vi "Heater Main PID.vi"() -> ()   [LabVIEW 2019]
doc: "This example demonstrates how to acquire a continuous amount of data (Waveform) using the DAQ device's internal clock. It also shows how to synchronize two devices for different device families (E Series, S Series, M Series, X Series, DSA, and SC Express), to simultaneously acquire the data.\n\nFor instructions on how to connect your signals to the DAQ device, refer to your device documentation."
uses:
  <vilib>/Utility/error.llb/DialogType.ctl
  <vilib>/DAQmx/write.llb/DAQmx Write (Analog DBL 1Chan 1Samp).vi
  <vilib>/DAQmx/read.llb/DAQmx Read (Analog 1D Wfm NChan NSamp).vi
  <vilib>/DAQmx/configure/timing.llb/DAQmx Timing (Sample Clock).vi
  <vilib>/DAQmx/miscellaneous.llb/DAQmx Fill In Error Info.vi
  <vilib>/addons/control/pid/pid.llb/PID (DBL).vi
  <vilib>/addons/control/pid/NI_PID_pid.lvlib
panel:
  in  "Microhotplate Logger":T1(tab)
  in  "Stop":bool
  in  "Enable logging":bool caption="Enable"
  in  "File config":T2={"Filepath"=path "C:/Users/Administrator/Desktop/DAQ Heater Control/Test data", "Test ID"="test", "PC"="69DTQV2"}
  in  "Sampling config":cluster{"Fs":dbl, "#s":dbl}={"Fs"=1000.0, "#s"=1000.0} {"Fs" format="%.2p"}
  out "Logging":bool=TRUE
  in  "Output channel config":T3={"Output channel"="Dev1/ao0", "name to assign"="Heater Voltage"}
  in  "Voltage output limit":dbl=3.0 caption="Amplitude"
  in  "Current channel config":T4={"Channel Index"=1, "Shunt resistance"=10.0, "Channel name"="Heater Current"} {"Shunt resistance" format="%.4f"}
  in  "IV channel config":T5={"Voltage channel index"=0, "Current channel index"=2}
  out "IV channel names":T6={"Voltage channel name"="Heater Voltage", "Current channel name"="Heater Current"}
  in  "TCR config":T7={"TCR1"=0.00205, "TCR2"=3e-07, "TRH"=0.766, "TRM"=0.928} {"TRM" format="%.3f"; "TRH" format="%.3f"; "TCR2" format="%.2e"; "TCR1" format="%.2e"}
  in  "Ramb config":cluster{"Tamb":dbl, "Ramb":dbl}={"Tamb"=25.0, "Ramb"=39.041} {"Ramb" format="%.3f"; "Tamb" format="%.3f"}
  out "Shunt channel name":string="Heater Shunt"
  in  "Auto":bool=TRUE
  out "PID output":dbl=1.0846342997266931
  in  "output range":cluster{"output high":dbl, "output low":dbl}={"output high"=1.5, "output low"=0.0}
  in  "setpoint":dbl=50.0
  in  "PID gains":T8={"proportional gain (Kc)"=0.0005, "integral time (Ti, min)"=0.001, "derivative time (Td, min)"=5e-10} {"derivative time (Td, min)" format="%#.6g"; "integral time (Ti, min)" format="%#.6g"; "proportional gain (Kc)" format="%#.6g"}
  in  "reinitialize? (F)":bool
  in  "Heater voltage":dbl=1.0 caption="Amplitude"
  out "Heater shunt":dynamicdata(graph)=[{"t0"=timestamp(3666105535.7382436 s since 1904-01-01), "dt"=0.001, "Y"=[1.045682721640953], "attributes"=variant("NI_ChannelName"=variant(string "Heater Voltage (DC Voltage)"), "NI_OriginalChannelName"=variant(string "Heater Voltage"), "NI_UnitDescription"=variant(string "Volts"))}, {"t0"=timestamp(3666105535.7382545 s since 1904-01-01), "dt"=0.001, "Y"=[0.20913177965876184], "attributes"=variant("NI_ChannelName"=variant(string "Heater Shunt (DC Voltage)"), "NI_OriginalChannelName"=variant(string "Heater Shunt"), "NI_UnitDescription"=variant(string "Volts"))}, {"t0"=timestamp(3666105535.7382545 s since 1904-01-01), "dt"=0.001, "Y"=[0.02091317796587617], "attributes"=variant("NI_ChannelName"=variant(string "Heater Current (DC Voltage)"), "NI_OriginalChannelName"=variant(string "Heater Current"), "NI_UnitDescription"=variant(string "A"))}, {"t0"=timestamp(3666105535.7382436 s since 1904-01-01), "dt"=0.001, "Y"=[50.00114171697651], "attributes"=variant("NI_ChannelName"=variant(string "Heater Resistance (DC Voltage)"), "NI_OriginalChannelName"=variant(string "Heater Resistance"), "NI_UnitDescription"=variant(string "Ohms"))}, {"t0"=timestamp(3666105535.7382436 s since 1904-01-01), "dt"=0.001, "Y"=[0.021868549543891273], "attributes"=variant("NI_ChannelName"=variant(string "Heater Power (DC Voltage)"), "NI_OriginalChannelName"=variant(string "Heater Power"), "NI_UnitDescription"=variant(string "Ohms"))}, {"t0"=timestamp(3666105535.7382436 s since 1904-01-01), "dt"=0.001, "Y"=[187.06189603218616], "attributes"=variant("NI_ChannelName"=variant(string "Heater Temp (DC Voltage)"), "NI_OriginalChannelName"=variant(string "Heater Temp"), "NI_UnitDescription"=variant(string "degC"))}]
  out "Heater temperature":dynamicdata(graph)=[{"t0"=timestamp(3666105535.7382436 s since 1904-01-01), "dt"=0.001, "Y"=[1.045682721640953], "attributes"=variant("NI_ChannelName"=variant(string "Heater Voltage (DC Voltage)"), "NI_OriginalChannelName"=variant(string "Heater Voltage"), "NI_UnitDescription"=variant(string "Volts"))}, {"t0"=timestamp(3666105535.7382545 s since 1904-01-01), "dt"=0.001, "Y"=[0.20913177965876184], "attributes"=variant("NI_ChannelName"=variant(string "Heater Shunt (DC Voltage)"), "NI_OriginalChannelName"=variant(string "Heater Shunt"), "NI_UnitDescription"=variant(string "Volts"))}, {"t0"=timestamp(3666105535.7382545 s since 1904-01-01), "dt"=0.001, "Y"=[0.02091317796587617], "attributes"=variant("NI_ChannelName"=variant(string "Heater Current (DC Voltage)"), "NI_OriginalChannelName"=variant(string "Heater Current"), "NI_UnitDescription"=variant(string "A"))}, {"t0"=timestamp(3666105535.7382436 s since 1904-01-01), "dt"=0.001, "Y"=[50.00114171697651], "attributes"=variant("NI_ChannelName"=variant(string "Heater Resistance (DC Voltage)"), "NI_OriginalChannelName"=variant(string "Heater Resistance"), "NI_UnitDescription"=variant(string "Ohms"))}, {"t0"=timestamp(3666105535.7382436 s since 1904-01-01), "dt"=0.001, "Y"=[0.021868549543891273], "attributes"=variant("NI_ChannelName"=variant(string "Heater Power (DC Voltage)"), "NI_OriginalChannelName"=variant(string "Heater Power"), "NI_UnitDescription"=variant(string "Ohms"))}, {"t0"=timestamp(3666105535.7382436 s since 1904-01-01), "dt"=0.001, "Y"=[187.06189603218616], "attributes"=variant("NI_ChannelName"=variant(string "Heater Temp (DC Voltage)"), "NI_OriginalChannelName"=variant(string "Heater Temp"), "NI_UnitDescription"=variant(string "degC"))}]
  out "Heater current":dynamicdata(graph)=[{"t0"=timestamp(3666105535.7382436 s since 1904-01-01), "dt"=0.001, "Y"=[1.045682721640953], "attributes"=variant("NI_ChannelName"=variant(string "Heater Voltage (DC Voltage)"), "NI_OriginalChannelName"=variant(string "Heater Voltage"), "NI_UnitDescription"=variant(string "Volts"))}, {"t0"=timestamp(3666105535.7382545 s since 1904-01-01), "dt"=0.001, "Y"=[0.20913177965876184], "attributes"=variant("NI_ChannelName"=variant(string "Heater Shunt (DC Voltage)"), "NI_OriginalChannelName"=variant(string "Heater Shunt"), "NI_UnitDescription"=variant(string "Volts"))}, {"t0"=timestamp(3666105535.7382545 s since 1904-01-01), "dt"=0.001, "Y"=[0.02091317796587617], "attributes"=variant("NI_ChannelName"=variant(string "Heater Current (DC Voltage)"), "NI_OriginalChannelName"=variant(string "Heater Current"), "NI_UnitDescription"=variant(string "A"))}, {"t0"=timestamp(3666105535.7382436 s since 1904-01-01), "dt"=0.001, "Y"=[50.00114171697651], "attributes"=variant("NI_ChannelName"=variant(string "Heater Resistance (DC Voltage)"), "NI_OriginalChannelName"=variant(string "Heater Resistance"), "NI_UnitDescription"=variant(string "Ohms"))}, {"t0"=timestamp(3666105535.7382436 s since 1904-01-01), "dt"=0.001, "Y"=[0.021868549543891273], "attributes"=variant("NI_ChannelName"=variant(string "Heater Power (DC Voltage)"), "NI_OriginalChannelName"=variant(string "Heater Power"), "NI_UnitDescription"=variant(string "Ohms"))}, {"t0"=timestamp(3666105535.7382436 s since 1904-01-01), "dt"=0.001, "Y"=[187.06189603218616], "attributes"=variant("NI_ChannelName"=variant(string "Heater Temp (DC Voltage)"), "NI_OriginalChannelName"=variant(string "Heater Temp"), "NI_UnitDescription"=variant(string "degC"))}]
  out "Heater voltage":dynamicdata(graph)=[{"t0"=timestamp(3666105535.7382436 s since 1904-01-01), "dt"=0.001, "Y"=[1.045682721640953], "attributes"=variant("NI_ChannelName"=variant(string "Heater Voltage (DC Voltage)"), "NI_OriginalChannelName"=variant(string "Heater Voltage"), "NI_UnitDescription"=variant(string "Volts"))}, {"t0"=timestamp(3666105535.7382545 s since 1904-01-01), "dt"=0.001, "Y"=[0.20913177965876184], "attributes"=variant("NI_ChannelName"=variant(string "Heater Shunt (DC Voltage)"), "NI_OriginalChannelName"=variant(string "Heater Shunt"), "NI_UnitDescription"=variant(string "Volts"))}, {"t0"=timestamp(3666105535.7382545 s since 1904-01-01), "dt"=0.001, "Y"=[0.02091317796587617], "attributes"=variant("NI_ChannelName"=variant(string "Heater Current (DC Voltage)"), "NI_OriginalChannelName"=variant(string "Heater Current"), "NI_UnitDescription"=variant(string "A"))}, {"t0"=timestamp(3666105535.7382436 s since 1904-01-01), "dt"=0.001, "Y"=[50.00114171697651], "attributes"=variant("NI_ChannelName"=variant(string "Heater Resistance (DC Voltage)"), "NI_OriginalChannelName"=variant(string "Heater Resistance"), "NI_UnitDescription"=variant(string "Ohms"))}, {"t0"=timestamp(3666105535.7382436 s since 1904-01-01), "dt"=0.001, "Y"=[0.021868549543891273], "attributes"=variant("NI_ChannelName"=variant(string "Heater Power (DC Voltage)"), "NI_OriginalChannelName"=variant(string "Heater Power"), "NI_UnitDescription"=variant(string "Ohms"))}, {"t0"=timestamp(3666105535.7382436 s since 1904-01-01), "dt"=0.001, "Y"=[187.06189603218616], "attributes"=variant("NI_ChannelName"=variant(string "Heater Temp (DC Voltage)"), "NI_OriginalChannelName"=variant(string "Heater Temp"), "NI_UnitDescription"=variant(string "degC"))}]
  out "Heater resistance":dynamicdata(graph)=[{"t0"=timestamp(3666105535.7382436 s since 1904-01-01), "dt"=0.001, "Y"=[1.045682721640953], "attributes"=variant("NI_ChannelName"=variant(string "Heater Voltage (DC Voltage)"), "NI_OriginalChannelName"=variant(string "Heater Voltage"), "NI_UnitDescription"=variant(string "Volts"))}, {"t0"=timestamp(3666105535.7382545 s since 1904-01-01), "dt"=0.001, "Y"=[0.20913177965876184], "attributes"=variant("NI_ChannelName"=variant(string "Heater Shunt (DC Voltage)"), "NI_OriginalChannelName"=variant(string "Heater Shunt"), "NI_UnitDescription"=variant(string "Volts"))}, {"t0"=timestamp(3666105535.7382545 s since 1904-01-01), "dt"=0.001, "Y"=[0.02091317796587617], "attributes"=variant("NI_ChannelName"=variant(string "Heater Current (DC Voltage)"), "NI_OriginalChannelName"=variant(string "Heater Current"), "NI_UnitDescription"=variant(string "A"))}, {"t0"=timestamp(3666105535.7382436 s since 1904-01-01), "dt"=0.001, "Y"=[50.00114171697651], "attributes"=variant("NI_ChannelName"=variant(string "Heater Resistance (DC Voltage)"), "NI_OriginalChannelName"=variant(string "Heater Resistance"), "NI_UnitDescription"=variant(string "Ohms"))}, {"t0"=timestamp(3666105535.7382436 s since 1904-01-01), "dt"=0.001, "Y"=[0.021868549543891273], "attributes"=variant("NI_ChannelName"=variant(string "Heater Power (DC Voltage)"), "NI_OriginalChannelName"=variant(string "Heater Power"), "NI_UnitDescription"=variant(string "Ohms"))}, {"t0"=timestamp(3666105535.7382436 s since 1904-01-01), "dt"=0.001, "Y"=[187.06189603218616], "attributes"=variant("NI_ChannelName"=variant(string "Heater Temp (DC Voltage)"), "NI_OriginalChannelName"=variant(string "Heater Temp"), "NI_UnitDescription"=variant(string "degC"))}]
  in  "Channel 2 config":T9={"Channel"="Dev1/ai3", "Vmax"=1.0, "Vmin"=0.0, "name to assign"="Heater Shunt", "input terminal configuration"=10106} {"input terminal configuration" items=["Default"=-1, "RSE"=10083, "NRSE"=10078, "Differential"=10106, "Pseudodifferential"=12529]; "Vmin" format="%0.2f"; "Vmax" format="%0.2f"}
  in  "Channel 1 config":T9={"Channel"="Dev1/ai2", "Vmax"=2.0, "Vmin"=0.0, "name to assign"="Heater Voltage", "input terminal configuration"=10106} {"input terminal configuration" items=["Default"=-1, "RSE"=10083, "NRSE"=10078, "Differential"=10106, "Pseudodifferential"=12529]; "Vmin" format="%0.2f"; "Vmax" format="%0.2f"}
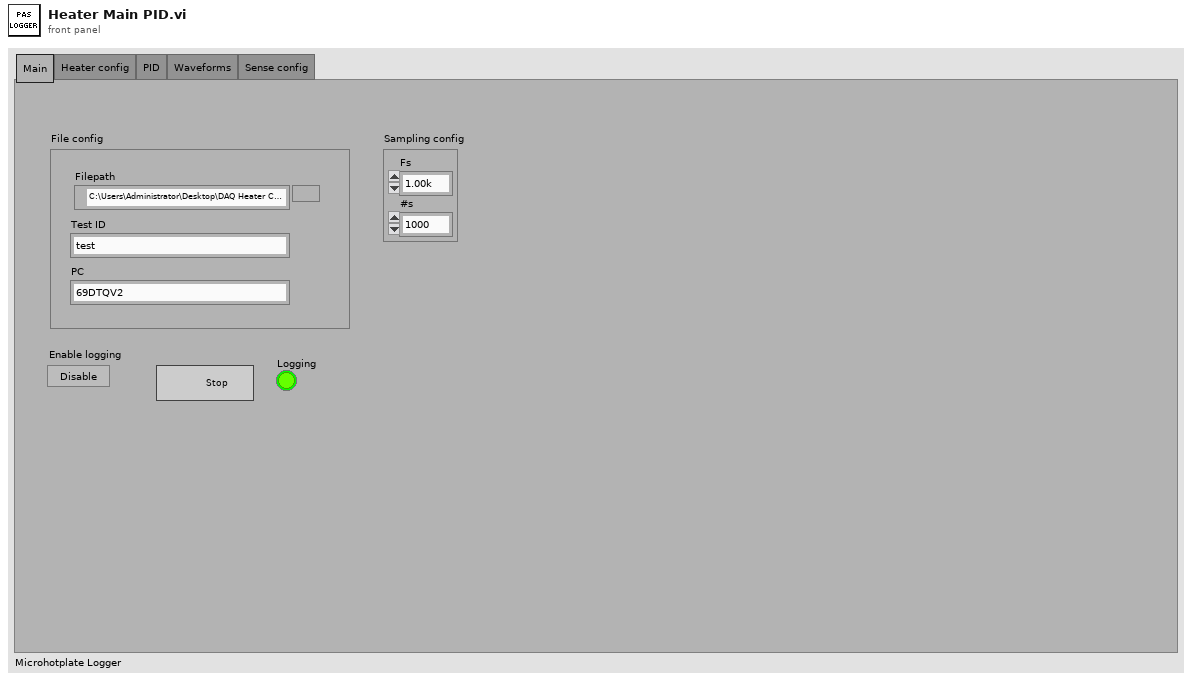
[diagram p1: front panel]
types:
  T1 = enum32{"Main", "Heater config", "PID", "Waveforms", "Sense config"}
  T2 = cluster{"Filepath":path, "Test ID":string, "PC":string}
  T3 = cluster{"Output channel":tag, "name to assign":string}
  T4 = cluster{"Channel Index":i32, "Shunt resistance":dbl, "Channel name":string}
  T5 = cluster{"Voltage channel index":i32, "Current channel index":i32}
  T6 = cluster{"Voltage channel name":string, "Current channel name":string}
  T7 = cluster{"TCR1":dbl, "TCR2":dbl, "TRH":dbl, "TRM":dbl}
  T8 = cluster{"proportional gain (Kc)":dbl, "integral time (Ti, min)":dbl, "derivative time (Td, min)":dbl}
  T9 = cluster{"Channel":tag, "Vmax":dbl, "Vmin":dbl, "name to assign":string, "input terminal configuration":i32}
  T10 = typedef "DialogType.ctl" = u16
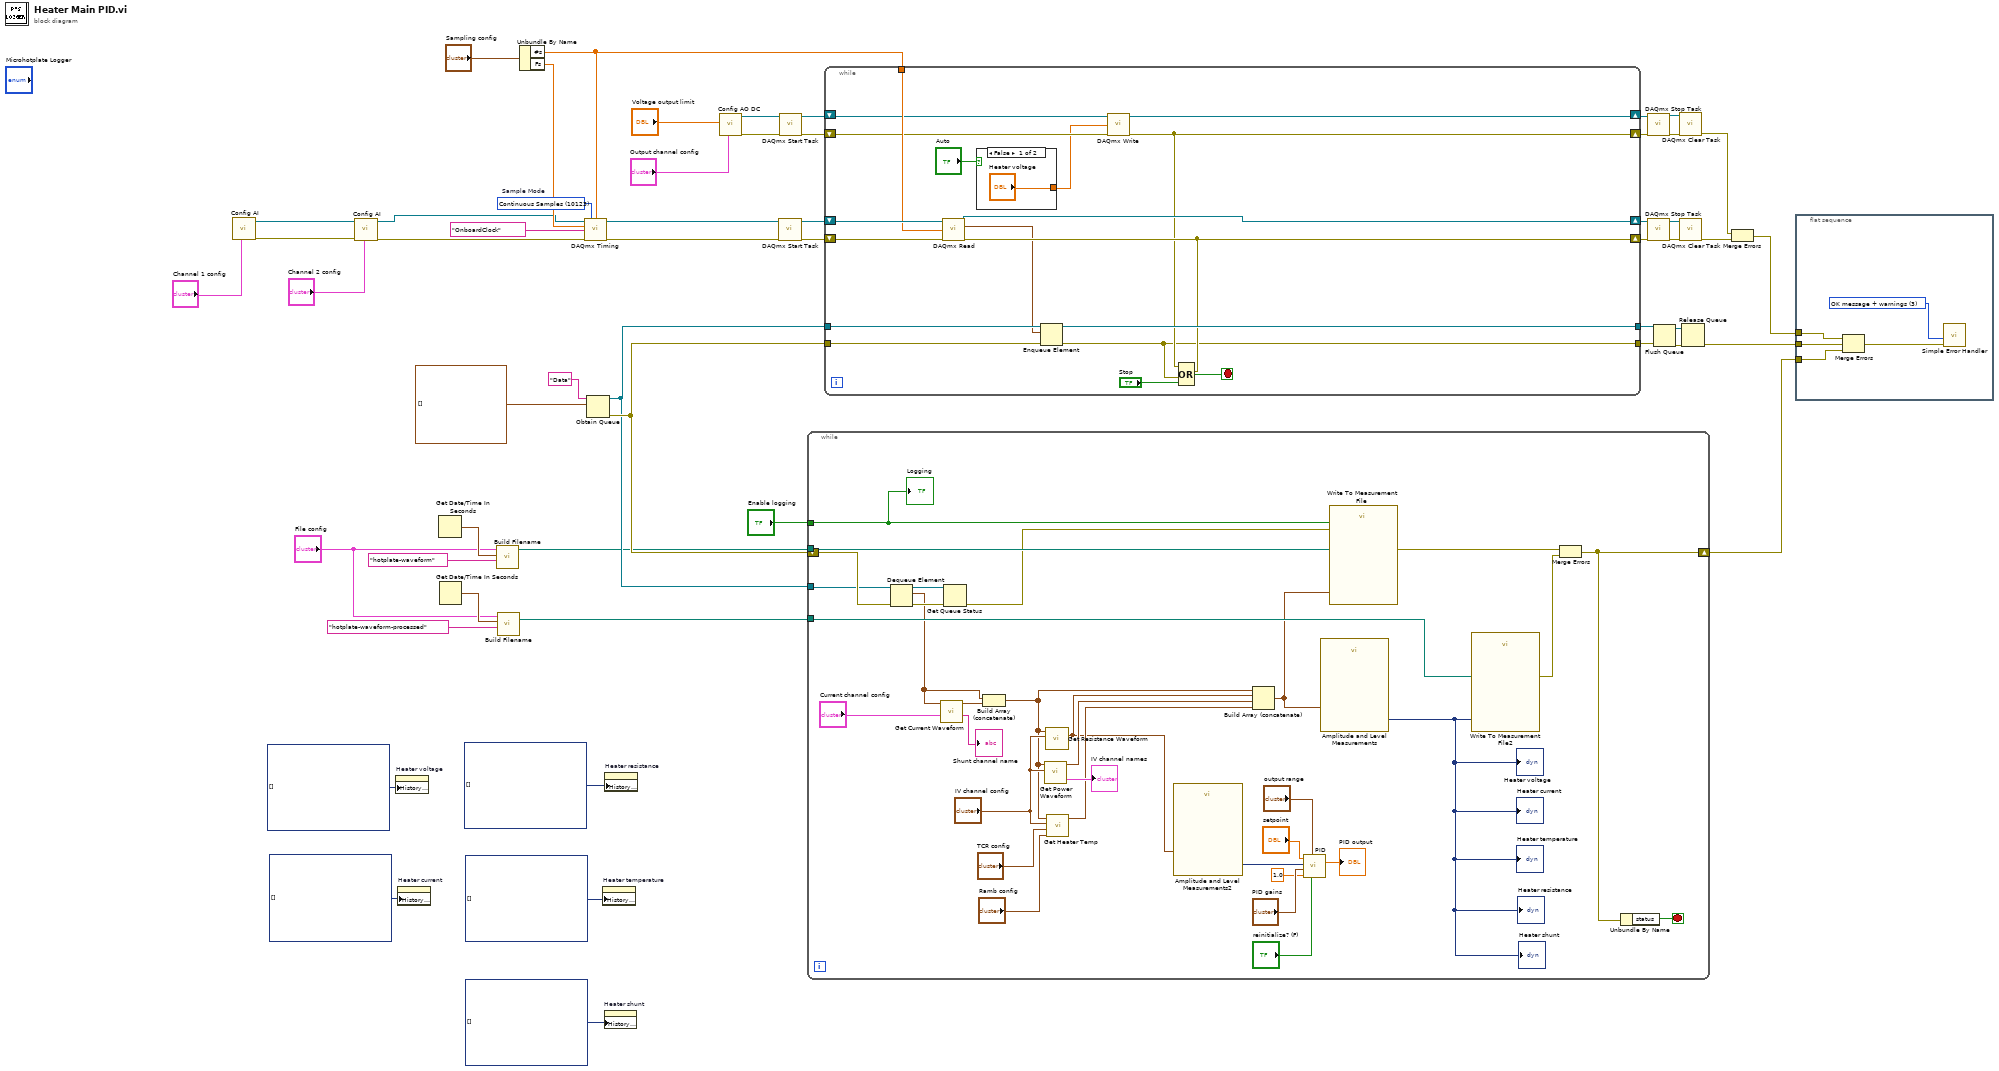
[diagram p0: block diagram]
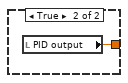
[diagram p2: hidden frame]
diagram:
  w45 = 10123 items=["Finite Samples"=10178, "Continuous Samples"=10123, "Hardware Timed Single Point"=12522]  # Sample Mode
  n1 = call "Config AI.vi"("Channel config"="Channel 1 config") -> ("error out"=w26:errorcluster, "task out"=w25:refnum<k21>)  [unwired: 9 in]
  n2 = call "Config AI.vi"("Channel config"="Channel 2 config", "error in"=w26, "task in"=w25) -> ("error out"=w4:errorcluster, "task out"=w3:refnum<k21>)  [unwired: 7 in]
  n3 = property on="Heater voltage" class="WFChart (strict)"("History Data"=dynamicdata[] []) -> ()  [unwired: 2 in, 2 out]
  n4 = property on="Heater current" class="WFChart (strict)"("History Data"=dynamicdata[] []) -> ()  [unwired: 2 in, 2 out]
  n5 = Get Date/Time In Seconds() -> (seconds since 1Jan1904=w19:timestamp)
  n6 = Get Date/Time In Seconds() -> (seconds since 1Jan1904=w14:timestamp)
  n7 = call "Build Filename.vi"("Test type"="hotplate-waveform" ("File type"), "time stamp"=w19, "File config"="File config") -> ("appended path"=w21:path)  [unwired: 8 in]
  n8 = call "Build Filename.vi"("Test type"="hotplate-waveform-processed" ("File type"), "time stamp"=w14, "File config"="File config") -> ("appended path"=w13:path)  [unwired: 8 in]
  n9 = Unbundle By Name("Sampling config") -> ("#s"=w6:dbl, "Fs"=w5:dbl)
  n10 = call-poly <vilib>:"DAQmx Timing.vi"("task/channels in"=w3, "sample mode"=w45, "samples per channel"=w6, "rate"=w5, "source"=tag "OnboardClock", "error in"=w4) -> ("task out"=w11:refnum<k21>, "error out"=w10:errorcluster)  [unwired: 8 in]
  n11 = Obtain Queue(name (unnamed)="Data" ("名前（名前なし）"), element data type=waveform(dbl)[] [] ("data")) -> (queue out=w29:refnum<queue>, error out=w30:errorcluster)  [unwired: 3 in, 1 out]
  n12 = property on="Heater temperature" class="WFChart (strict)"("History Data"=dynamicdata[] []) -> ()  [unwired: 2 in, 2 out]
  n13 = property on="Heater shunt" class="WFChart (strict)"("History Data"=dynamicdata[] []) -> ()  [unwired: 2 in, 2 out]
  n14 = property on="Heater resistance" class="WFChart (strict)"("History Data"=dynamicdata[] []) -> ()  [unwired: 2 in, 2 out]
  n15 = call "Config AO DC.vi"("Channel config"="Output channel config", "Voltage"="Voltage output limit") -> ("error out"=w39:errorcluster, "task out"=w40:refnum<k21>)  [unwired: 8 in]
  n16 = call <vilib>:"DAQmx Start Task.vi"("task/channels in"=w11, "error in"=w10) -> ("task out"=w41:refnum<k21>, "error out"=w42:errorcluster)  [unwired: 12 in]
  n17 = call <vilib>:"DAQmx Start Task.vi"("task/channels in"=w40, "error in"=w39) -> ("task out"=w43:refnum<k21>, "error out"=w44:errorcluster)  [unwired: 12 in]
  n18 = while {
    tunnel: w29 -> [w87]
    shift-right: [w80] -> w28
    shift-left: w30 -> [w88]
    tunnel: w21 -> [w86]
    tunnel: "Enable logging" -> [w82]
    tunnel: w13 -> [w77]
    stop <- w79 stop-if-true
    n19 = Dequeue Element(queue=w87, error in (no error)=w88) -> (queue out=w84:refnum<queue>, element=w68:waveform(dbl)[], error out=w85:errorcluster)  [unwired: 1 in, 1 out]
    n20 = call "Get Current Waveform.vi"("Config"="Current channel config", "array"=w68) -> ("Channel name"=→"Shunt channel name":string, "Current waveform out"=w74:waveform(dbl))  [unwired: 8 in]
    n21 = Get Queue Status(queue=w84, error in (no error)=w85) -> (error out=w83:errorcluster)  [unwired: 1 in, 7 out]
    n22 = Build Array (concatenate)(w68, w74) -> (w66:waveform(dbl)[])
    n23 = call "Get Power Waveform.vi"("Channel config"="IV channel config", "array"=w66) -> ("Power waveform out"=w69:waveform(dbl), "Channel names"=→"IV channel names":T6)  [unwired: 8 in]
    n24 = call "Get Resistance Waveform.vi"("Channel config"="IV channel config", "array"=w66) -> ("Resistance waveform out"=w58:waveform(dbl))  [unwired: 8 in, 1 out]
    n25 = call "Get Heater Temp.vi"("Ramb config"="Ramb config", "TCR config"="TCR config", "Channel config"="IV channel config", "array"=w66) -> ("waveform out"=w65:waveform(dbl))  [unwired: 6 in, 1 out]
    n26 = call "Amplitude and Level Measurements2"("Signals"=w58) -> ("Mean (DC)"=w60:dynamicdata)  [unwired: 13 in, 1 out]
    n27 = Build Array (concatenate)(w66, w58, w69, w65) -> (w76:waveform(dbl)[])
    n28 = call-poly <vilib>:"PID.vi"("reinitialize? (F)"="reinitialize? (F)", "output range"="output range", "dt (s)"=1.0, "PID gains"="PID gains", "process variable"=w60, "setpoint"="setpoint") -> ("output"=→"PID output":dbl)  [unwired: 4 in, 1 out]
    n29 = call "Amplitude and Level Measurements"("Signals"=w76) -> ("Mean (DC)"=w67:dynamicdata)  [unwired: 13 in, 1 out]
    "Heater voltage" <- w67
    "Heater current" <- w67
    "Heater temperature" <- w67
    "Heater resistance" <- w67
    "Heater shunt" <- w67
    n30 = call "Write To Measurement File"("Signals"=w76, "Enable"=w82, "error in (no error)"=w83, "Filename"=w86) -> ("error out"=w81:errorcluster)  [unwired: 13 in, 2 out]
    n31 = call "Write To Measurement File2"("Signals"=w67, "Filename"=w77) -> ("error out"=w78:errorcluster)  [unwired: 15 in, 2 out]
    n32 = Merge Errors(w81, w78) -> (w80:errorcluster)
    n33 = Unbundle By Name(w80) -> ("status"=w79:bool)
    "Logging" <- w82
  }
  n34 = while {
    shift-right: [w94] -> w54
    shift-left: w44 -> [w95]
    shift-right: [w97] -> w50
    shift-left: w42 -> [w104]
    shift-right: [w92] -> w55
    shift-left: w43 -> [w93]
    shift-right: [w103] -> w51
    shift-left: w41 -> [w105]
    tunnel: w6 -> [w102]
    tunnel: [w101] -> w35
    tunnel: [w91] -> w34
    tunnel: w29 -> [w100]
    tunnel: w30 -> [w99]
    stop <- w106 stop-if-true
    n35 = call-poly <vilib>:"DAQmx Read.vi"("task/channels in"=w105, "number of samples per channel"=w102, "error in"=w104) -> ("task out"=w103:refnum<k21>, "data"=w96:waveform(dbl)[], "error out"=w97:errorcluster)  [unwired: 10 in]
    n36 = case shown="False" "Auto" {
      tunnel: ["Heater voltage" w108] -> w89
      frame False {
      }
      frame True {
        n37 = local read "PID output"() -> (w108:dbl)
      }
    }
    n38 = Enqueue Element(queue=w100, element=w96, error in (no error)=w99) -> (queue out=w101:refnum<queue>, error out=w91:errorcluster)  [unwired: 1 in, 1 out]
    n39 = call-poly <vilib>:"DAQmx Write.vi"("task/channels in"=w93, "data"=w89, "error in"=w95) -> ("task out"=w92:refnum<k21>, "error out"=w94:errorcluster)  [unwired: 10 in, 1 out]
    n40 = Compound Arithmetic op=OR(w94, w97, w91, "Stop") -> (w106:bool)
  }
  n41 = call <vilib>:"DAQmx Stop Task.vi"("task/channels in"=w55, "error in"=w54) -> ("task out"=w52:refnum<k21>, "error out"=w53:errorcluster)  [unwired: 12 in]
  n42 = call <vilib>:"DAQmx Stop Task.vi"("task/channels in"=w51, "error in"=w50) -> ("task out"=w48:refnum<k21>, "error out"=w49:errorcluster)  [unwired: 12 in]
  n43 = Flush Queue(queue=w35, error in (no error)=w34) -> (queue out=w36:refnum<queue>, error out=w37:errorcluster)  [unwired: 1 out]
  n44 = call <vilib>:"DAQmx Clear Task.vi"("task in"=w52, "error in"=w53) -> ("error out"=w47:errorcluster)  [unwired: 13 in]
  n45 = call <vilib>:"DAQmx Clear Task.vi"("task in"=w48, "error in"=w49) -> ("error out"=w46:errorcluster)  [unwired: 13 in]
  n46 = Release Queue(queue=w36, error in (no error)=w37) -> (error out=w32:errorcluster)  [unwired: 1 in, 2 out]
  n47 = Merge Errors(w47, w46) -> (w33:errorcluster)
  n48 = flat-sequence {
    tunnel: w33 -> [w113]
    tunnel: w32 -> [w112]
    tunnel: w28 -> [w109]
    frame #0 {
      w111 = T10 3 items=["no dialog", "OK message", "continue or stop message", "OK message + warnings", "continue/stop + warnings"] ("type of dialog (OK msg:1)")
      n49 = Merge Errors(w113, w112, w109) -> (w110:errorcluster)
      n50 = call <vilib>:"Simple Error Handler.vi"("type of dialog (OK msg:1)"=w111, "error in (no error)"=w110) -> ()  [unwired: 3 in, 5 out]
    }
  }
